vi "CheckVersion_Wiresmith.vi"() -> ()   [LabVIEW 2019]
uses:
  <vilib>/Wiresmith Technology/G CLI/CLI Class/CLI.lvclass
panel:
  out "Version to Match":string
  out "Matches Version":bool
  out "Version String":string
  out "Path to Scan":path
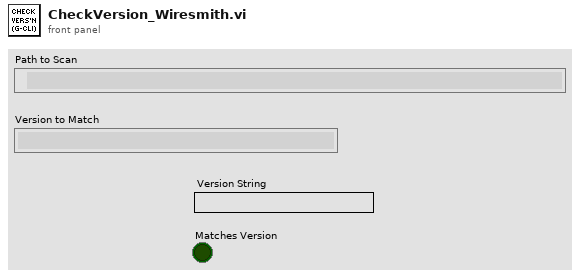
[diagram p1: front panel]
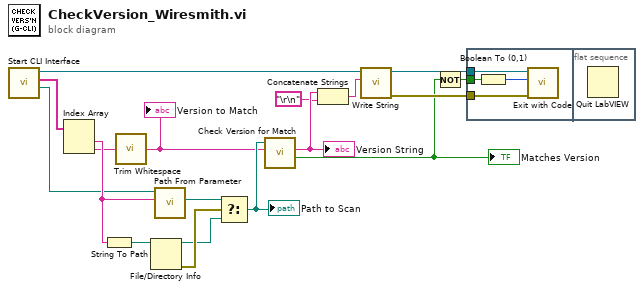
[diagram p0: block diagram]
diagram:
  n1 = call <vilib>:"Start CLI Interface.vi"() -> ("Working Directory"=w2:path, "Custom Parameters"=w14:string[], "CLI out"=w15:refnum<class "CLI.lvclass">)  [unwired: 8 in, 1 out]
  n2 = Index Array(array=w14) -> (element #1=w18:string, element #2=w13:string)  [unwired: 2 in]
  n3 = String To Path(string=w18) -> (path=w8:path)
  n4 = call <vilib>:"Trim Whitespace.vi"("string"=w13) -> ("trimmed string"=w4:string)  [unwired: 1 in]
  "Version to Match" <- w4
  n5 = File/Directory Info(path=w8) -> (path out=w9:path, error out=w10:errorcluster)  [unwired: 1 in, 5 out]
  n6 = call <vilib>:"Path From Parameter.vi"("Path Parameter"=w18, "Working Directory"=w2) -> ("Full Path"=w1:path)  [unwired: 9 in]
  n7 = Select(t=w1, s=w10, f=w9) -> (s? t:f=w7:path)
  "Path to Scan" <- w7
  n8 = call "Check Version for Match.vi"("Version to Match"=w4, "PPL Path"=w7) -> ("Matches Version"=w12:bool, "Version String"=w11:string)  [unwired: 8 in]
  "Version String" <- w11
  "Matches Version" <- w12
  n9 = Concatenate Strings(w11, "\r\n") -> (w6:string)
  n10 = call <vilib>:"Write String.vi"("Text to Write"=w6, "CLI in"=w15) -> ("error out"=w16:errorcluster, "CLI out"=w17:refnum<class "CLI.lvclass">)  [unwired: 8 in]
  n11 = Not(x=w12) -> (.not. x?=w3:bool)
  n12 = flat-sequence {
    tunnel: w17 -> [w21]
    tunnel: w16 -> [w20]
    tunnel: w3 -> [w19]
    frame #0 {
      n13 = Boolean To (0,1)(Boolean=w19) -> (0, 1=w22:i16)
      n14 = call <vilib>:"Exit with Code.vi"("error in (no error)"=w20, "Exit Code (0)"=w22, "CLI in"=w21) -> ()  [unwired: 8 in, 1 out]
    }
    frame #1 {
      n15 = Quit LabVIEW() -> ()  [unwired: 1 in]
    }
  }
